vi "Calculation result path.vi"(11 "Measurement path":path) -> (1 "file exists?":bool, 3 "calc result info path":path)   [LabVIEW 2020]
doc: "From measurement directory path, search for calculation result, and returns path of the info file with calculation result."
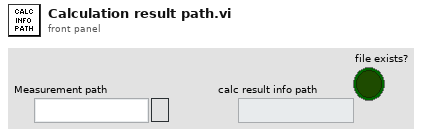
[diagram p1: front panel]
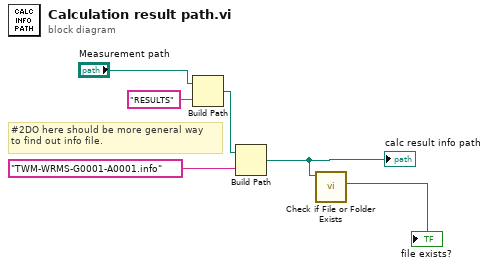
[diagram p0: block diagram]
diagram:
  # "#2DO here should be more general way\nto find out info file."
  n1 = Build Path(base path="Measurement path", name or relative path="RESULTS") -> (appended path=w4:path)
  n2 = Build Path(base path=w4, name or relative path="TWM-WRMS-G0001-A0001.info") -> (appended path=w2:path)
  "calc result info path" <- w2
  n3 = call <vilib>:"Check if File or Folder Exists.vi"("path"=w2) -> ("file or folder exists?"=→"file exists?":bool)  [unwired: 8 in, 2 out]
